vi "Pendiente de una recta.vi"() -> ()   [LabVIEW 2020]
panel:
  in  "String":string
  in  "stop":bool
  out "Cruce por cero (b)":dbl
  in  "X1":dbl
  in  "X2":dbl
  out "Pendiente":dbl
  in  "Y1":dbl
  in  "Y2":dbl
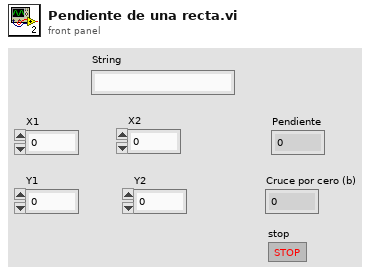
[diagram p1: front panel]
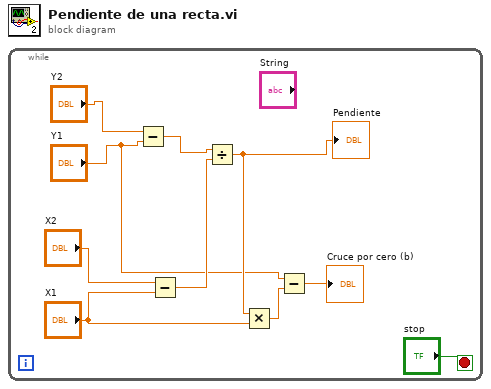
[diagram p0: block diagram]
diagram:
  n1 = while {
    stop <- "stop" stop-if-true
    n2 = Subtract(x="Y2", y="Y1") -> (x-y=w8:dbl)
    n3 = Subtract(x="X2", y="X1") -> (x-y=w7:dbl)
    n4 = Divide(x=w8, y=w7) -> (x/y=w5:dbl)
    "Pendiente" <- w5
    n5 = Multiply(x=w5, y="X1") -> (x*y=w4:dbl)
    n6 = Subtract(x="Y1", y=w4) -> (x-y=→"Cruce por cero (b)":dbl)
  }
